vi "testHeadersPresentParserSupport.vi"(8 "error in (no error)":errorcluster, 11 "reference in":refnum<class "EasyXMLTest.lvclass">) -> (0 "error out":errorcluster, 3 "reference in":refnum<class "EasyXMLTest.lvclass">)   [LabVIEW 2013, in "EasyXMLTest.lvclass"]
uses:
  EasyXMLTest.lvclass
panel:
  in  "a":cluster{"b":string}={"b"="1"}
  out "a":cluster{"b":string}
  in  "XML String":string="<?xml version=\"1.0\" standalone=\"yes\"?>\n<?xml-stylesheet type=\"text/xsl\" href=\"http://www.example.com/example.xsl\"?>\n<a>\n<b>1</b>\n</a>"
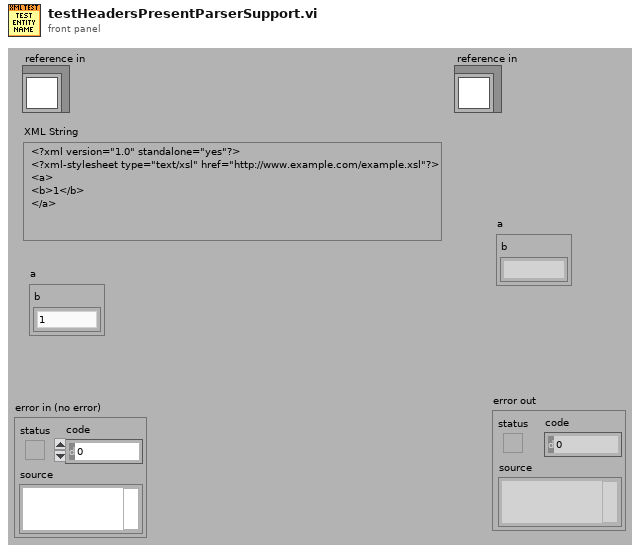
[diagram p1: front panel]
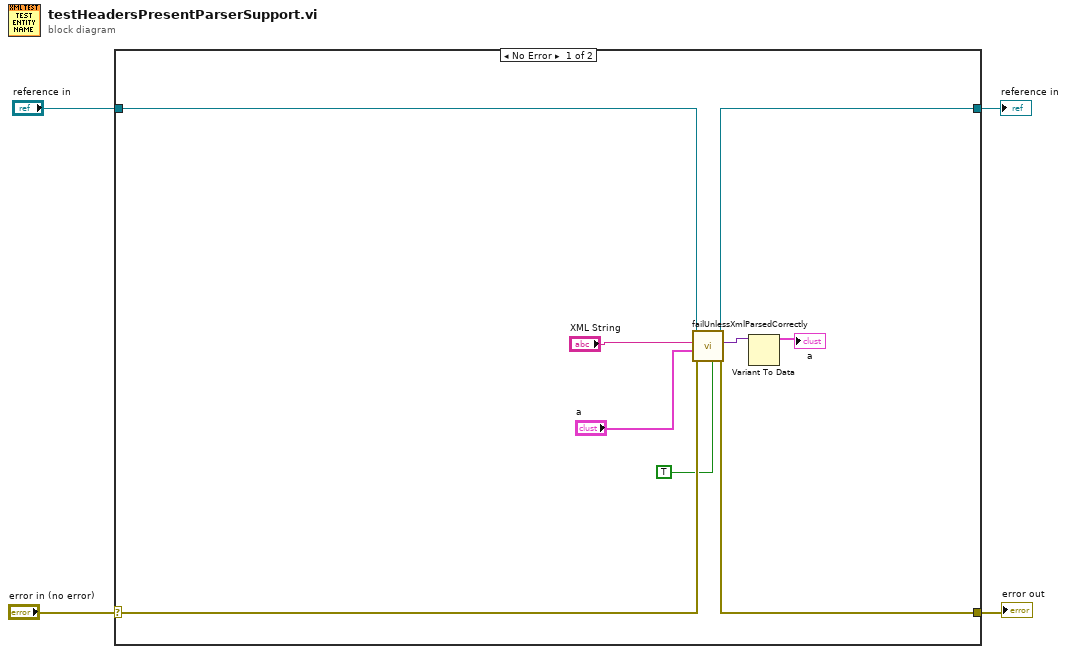
[diagram p0: block diagram]
diagram:
  n1 = case shown="No Error" "error in (no error)" {
    selector: "error in (no error)" -> [w11 w15]
    tunnel: [w6 w15] -> w3
    tunnel: [w12 w14] -> w1
    tunnel: "reference in" -> [w13 w14]
    frame No Error {
      n2 = call "failUnlessXmlParsedCorrectly.vi"("Convert EOL? (TRUE)"=TRUE, "error in"=w11, "Expected Data"="a", "XML String"="XML String", "reference in"=w13) -> ("error out"=w6:errorcluster, "Produced Data"=w9:variant, "reference in"=w12:refnum<class "EasyXMLTest.lvclass">)  [unwired: 4 in]
      n3 = Variant To Data(Variant=w9) -> (data=→"a":cluster{"b":string})  [unwired: 2 in, 1 out]
    }
    frame Error {
    }
  }
  "error out" <- w3
  "reference in" <- w1
